vi "Camera.GetSession.vi"(8 "error in (no error)":errorcluster, 11 "Camera.Simulated":refnum<class "Camera.IMAQdx.lvclass">) -> (0 "error out":errorcluster, 1 "Image":T1, 2 "Session":T2, 3 "Camera.Simulated":refnum<class "Camera.IMAQdx.lvclass">)   [LabVIEW 2015, in "Camera.IMAQdx.lvclass"]
doc: "---------------------------------------------------------------\nJKI State Machine Objects™\nhttp://jki.net/state-machine-objects/\nCopyright (C) 2005-2015, JKI <info@jki.net>\nALL RIGHTS RESERVEDJKI State Machine Objects (SMO) 1.0.0.5\nJKI - JKI\nCopyright (c) 2016, JKI"
uses:
  Camera.IMAQdx.lvclass
  <vilib>/userdefined/High Color/IMAQdx.ctl
  <vilib>/vision/Image Controls.llb/IMAQ Image.ctl
  Camera.IMAQdx.lvclass/Camera.IMAQdx.ctl
panel:
  # "For instructions on how to use the JKI State Machine Objects, examples and video tutorials, visit:\nhttp://jki.net/state-machine-objects/\n\nJKI State Machine Objects™\nhttp://jki.net/state-machine-objects/\nCopyright (C) 2005-2015, JKI <info@jki.net>\nALL RIGHTS RESERVED"
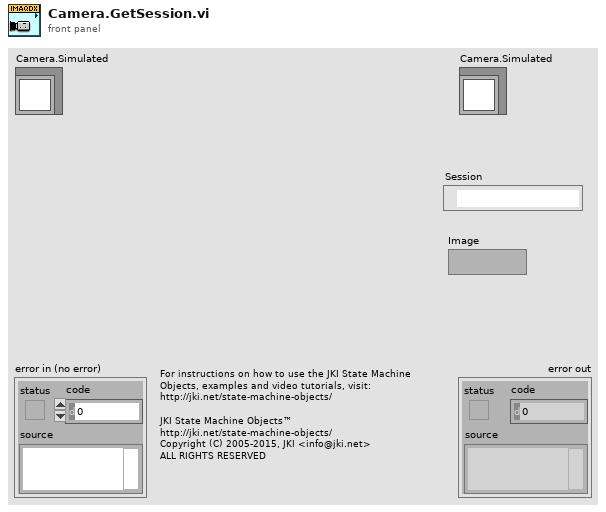
[diagram p1: front panel]
types:
  T1 = typedef "IMAQ Image.ctl" = refnum<image>
  T2 = typedef "IMAQdx.ctl" = refnum<k21>
  T3 = typedef "Camera.IMAQdx.lvclass/PrivateData--Ref.ctl" = refnum<data-value>
  T4 = typedef "Camera.IMAQdx.lvclass/PrivateData--Cluster.ctl" = cluster{"Session":T2, "Image":T1}
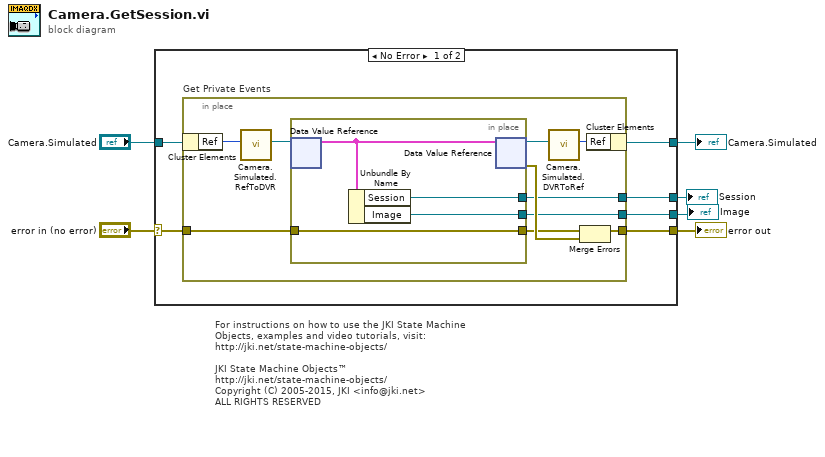
[diagram p0: block diagram]
diagram:
  # "For instructions on how to use the JKI State Machine Objects, examples and video tutorials, visit:\nhttp://jki.net/state-machine-objects/\n\nJKI State Machine Objects™\nhttp://jki.net/state-machine-objects/\nCopyright (C) 2005-2015, JKI <info@jki.net>\nALL RIGHTS RESERVED"
  n1 = case shown="No Error" "error in (no error)" {
    selector: "error in (no error)" -> [w11 w27]
    tunnel: "Camera.Simulated" -> [w12 w28]
    tunnel: [w10 w27] -> w5
    tunnel: [w9 w28] -> w4
    tunnel: [w8 _] -> w2
    tunnel: [w7 _] -> w1
    frame No Error {
      n2 = in-place "Get Private Events" {
        in-place-border: w11 -> [w22]
        in-place-border: [w19] -> w10
        in-place-border: [w18] -> w8
        in-place-border: [w13] -> w7
        n3 = in-place-cluster #1(w12) -> ("Ref"=w17:u32)
        n4 = call "Camera.Simulated.RefToDVR.vi"("Ref"=w17) -> ("Ref"=w16:T3)  [unwired: 10 in]
        n5 = in-place {
          in-place-border: w22 -> [w25]
          in-place-border: [w25] -> w20
          in-place-border: [w24] -> w18
          in-place-border: [w23] -> w13
          n6 = in-place-dvr #2(w16) -> (w26:T4)  [unwired: 1 out]
          n7 = Unbundle By Name(w26) -> ("Session"=w24:T2, "Image"=w23:T1)
          n8 = in-place-dvr #2(w26) -> (w15:T3, w21:errorcluster)
        }
        n9 = call "Camera.Simulated.DVRToRef.vi"("Ref"=w15) -> ("Ref"=w14:u32)  [unwired: 10 in]
        n10 = Merge Errors(w20, w21) -> (w19:errorcluster)
        n11 = in-place-cluster #1("Ref"=w14) -> (w9:refnum<class "Camera.IMAQdx.lvclass">)
      }
    }
    frame Error {
    }
  }
  "error out" <- w5
  "Camera.Simulated" <- w4
  "Session" <- w2
  "Image" <- w1
